vi "Mapping Math.vi"(4 "Distance Update in mm":i16, 5 "X Coordinate":dbl, 6 "Y Coordinate":dbl, 7 "Angle Update in degrees":i16, 8 "Pose in Radians":dbl) -> (0 "X out":dbl, 1 "Y out":dbl, 2 "Radius":dbl, 3 "Pose Out":dbl)   [LabVIEW 2010]
panel:
  out "Y center":dbl
  out "X center":dbl
  out "Angle update in radians":dbl
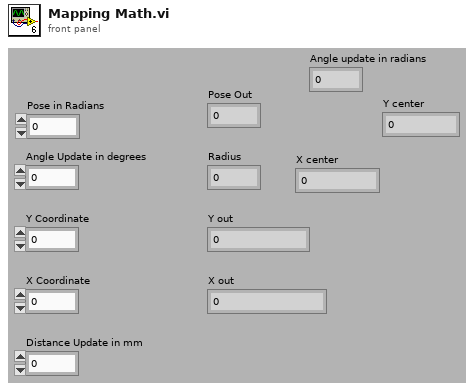
[diagram p1: front panel]
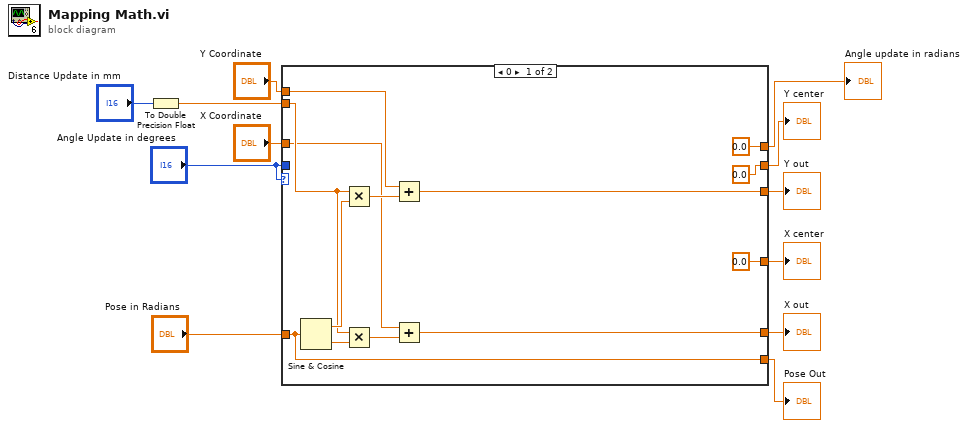
[diagram p0: block diagram]
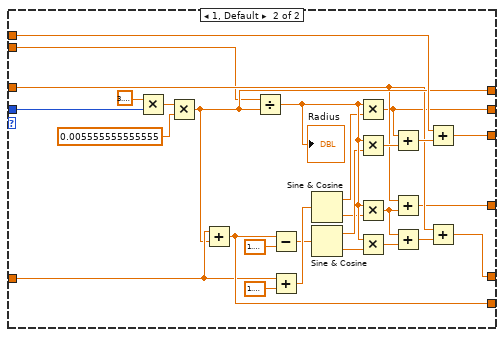
[diagram p2: hidden frame]
diagram:
  n1 = To Double Precision Float(number="Distance Update in mm") -> (double precision float=w1:dbl)
  n2 = case shown="0" "Angle Update in degrees" {
    tunnel: [w18 w53] -> w12
    tunnel: [w17 w52] -> w11
    tunnel: "Y Coordinate" -> [w20 w50]
    tunnel: [w14 w43] -> w9
    tunnel: "Pose in Radians" -> [w14 w39]
    tunnel: [0.0 w37] -> w7
    tunnel: "Angle Update in degrees" -> [_ w33]
    tunnel: "X Coordinate" -> [w19 w32]
    tunnel: [0.0 w30] -> w5
    tunnel: [0.0 w29] -> w4
    tunnel: w1 -> [w23 w26]
    frame 0 {
      n3 = Sine & Cosine(0:w14) -> (1:w24:dbl, 2:w25:dbl)
      n4 = Multiply(x=w23, y=w24) -> (x*y=w21:dbl)
      n5 = Multiply(x=w23, y=w25) -> (x*y=w22:dbl)
      n6 = Add(x=w20, y=w21) -> (x+y=w18:dbl)
      n7 = Add(x=w19, y=w22) -> (x+y=w17:dbl)
    }
    frame 1, Default {
      n8 = Multiply(x=3.141592653589793, y=w33) -> (x*y=w35:dbl)
      n9 = Multiply(x=w35, y=0.005555555555555) -> (x*y=w37:dbl)
      n10 = Add(x=w39, y=w37) -> (x+y=w43:dbl)
      n11 = Divide(x=w26, y=w37) -> (x/y=w46:dbl)
      "Radius" <- w46
      n12 = Subtract(x=w43, y=1.5707963267948966) -> (x-y=w28:dbl)
      n13 = Add(x=w39, y=1.5707963267948966) -> (x+y=w40:dbl)
      n14 = Sine & Cosine(0:w40) -> (1:w42:dbl, 2:w41:dbl)
      n15 = Sine & Cosine(0:w28) -> (1:w45:dbl, 2:w44:dbl)
      n16 = Multiply(x=w46, y=w42) -> (x*y=w29:dbl)
      n17 = Multiply(x=w46, y=w45) -> (x*y=w48:dbl)
      n18 = Multiply(x=w46, y=w41) -> (x*y=w31:dbl)
      n19 = Multiply(x=w46, y=w44) -> (x*y=w47:dbl)
      n20 = Add(x=w29, y=w48) -> (x+y=w49:dbl)
      n21 = Add(x=w32, y=w31) -> (x+y=w30:dbl)
      n22 = Add(x=w31, y=w47) -> (x+y=w51:dbl)
      n23 = Add(x=w50, y=w49) -> (x+y=w53:dbl)
      n24 = Add(x=w32, y=w51) -> (x+y=w52:dbl)
    }
  }
  "Y out" <- w12
  "X out" <- w11
  "Pose Out" <- w9
  "Angle update in radians" <- w7
  "X center" <- w5
  "Y center" <- w4
